vi "eFGV - Refresh IO.vi"(6 "States":T1, 8 "Error In":errorcluster, 11 "Refresh IO":bool) -> (0 "Error Out":errorcluster, 2 "Event Refresh IO":refnum<user-event>)   [LabVIEW 2020]
uses:
  Control/State - eFGV.ctl
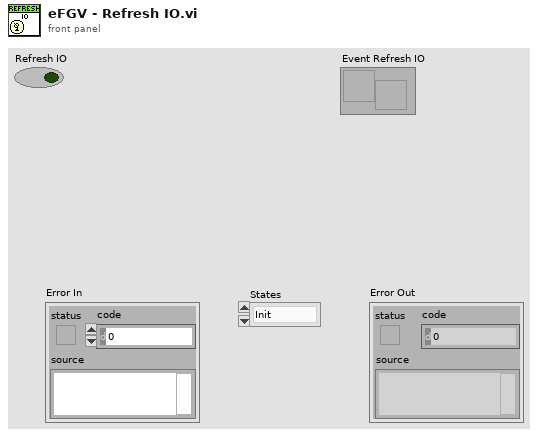
[diagram p1: front panel]
types:
  T1 = typedef "State - eFGV.ctl" = enum16{"Init", "Read", "Write", "Exit"}
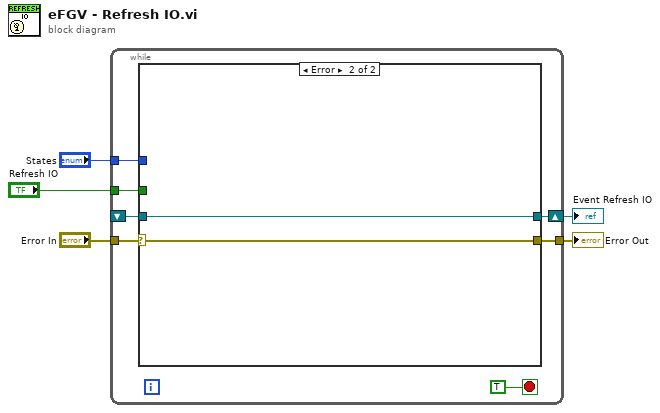
[diagram p0: block diagram]
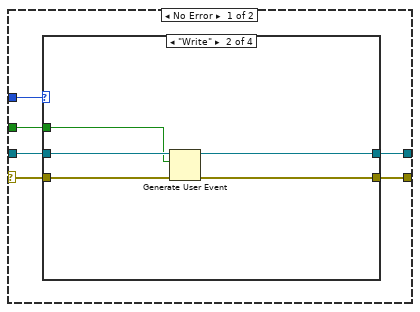
[diagram p2: hidden frame]
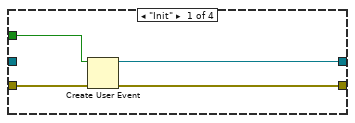
[diagram p3: hidden frame]
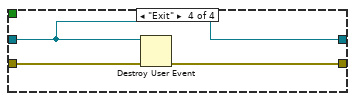
[diagram p5: hidden frame]
diagram:
  n1 = while {
    tunnel: "Error In" -> [w12]
    tunnel: [w11] -> w4
    tunnel: "States" -> [w9]
    shift-right: [w6] -> w1
    shift-left: _ -> [w8]
    tunnel: "Refresh IO" -> [w7]
    stop <- TRUE stop-if-true
    n2 = case shown="Error" w12 {
      selector: w12 -> [w18 w34]
      tunnel: [w17 w34] -> w11
      tunnel: w9 -> [w16 _]
      tunnel: w8 -> [w15 w33]
      tunnel: w7 -> [w14 _]
      tunnel: [w13 w33] -> w6
      frame No Error {
        n3 = case shown="\"Write\"" w16 {
          tunnel: w18 -> [w22 w27 w29 w32]
          tunnel: [w21 w26 w29 w31] -> w17
          tunnel: w15 -> [_ w25 w28 w30]
          tunnel: w14 -> [w20 w23 _ _]
          tunnel: [w19 w24 w28 w30] -> w13
          frame "Init" {
            n4 = Create User Event(user event datatype=w20, error in=w22) -> (user event=w19:refnum<user-event>, error out=w21:errorcluster)
          }
          frame "Write" {
            n5 = Generate User Event(user event=w25, event data cluster=w23, error in=w27) -> (user event out=w24:refnum<user-event>, error out=w26:errorcluster)  [unwired: 1 in]
          }
          frame "Read" {
          }
          frame "Exit" {
            n6 = Destroy User Event(user event=w30, error in=w32) -> (error out=w31:errorcluster)
          }
        }
      }
      frame Error {
      }
    }
  }
  "Error Out" <- w4
  "Event Refresh IO" <- w1
